vi "meth.PushClusterArray.vi"(0 "class.GLue in":refnum<class "class.GLue.lvclass">, 7 "Array":variant[](array[variant]), 11 "error in":errorcluster) -> (4 "class.GLue out":refnum<class "class.GLue.lvclass">, 8 "Pushed?":bool=TRUE, 15 "error out":errorcluster)   [LabVIEW 2014, in "GLue.lvlib" / "class.GLue.lvclass"]
uses:
  class.GLue.lvclass
  class.GLue.lvclass/class.GLue.ctl
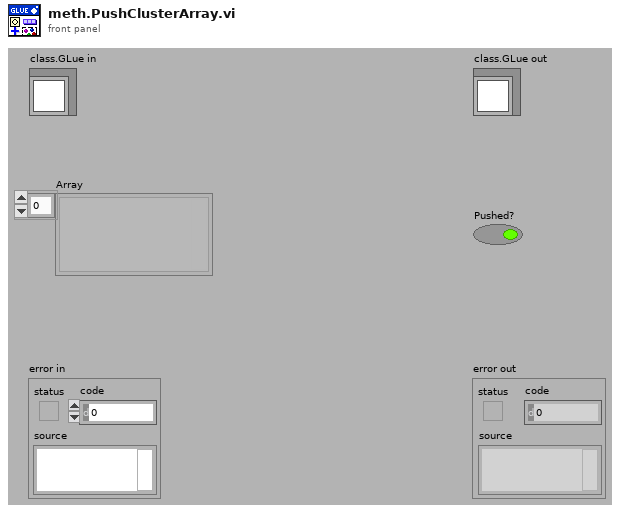
[diagram p1: front panel]
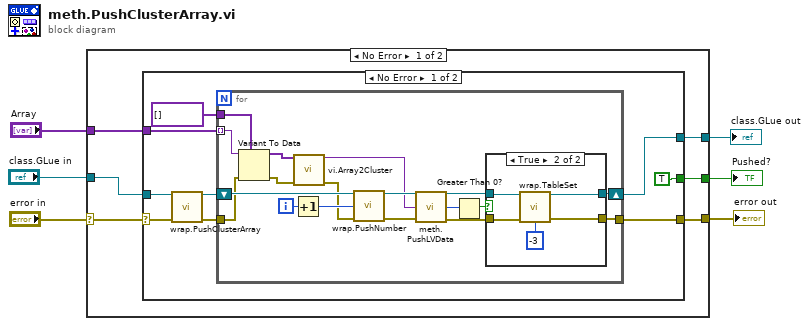
[diagram p0: block diagram]
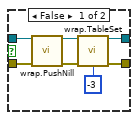
[diagram p2: hidden frame]
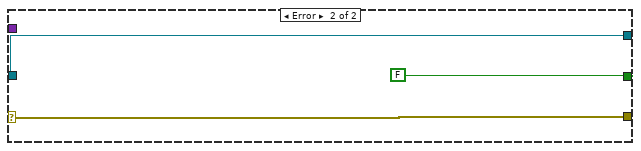
[diagram p4: hidden frame]
diagram:
  n1 = case shown="No Error" "error in" {
    selector: "error in" -> [w8 w57]
    tunnel: [w7 w57] -> w6
    tunnel: [w11 w56] -> w4
    tunnel: "class.GLue in" -> [w12 w56]
    tunnel: [w10 FALSE] -> w2
    tunnel: "Array" -> [w9 _]
    frame No Error {
      n2 = case shown="No Error" w8 {
        selector: w8 -> [w17 w54]
        tunnel: w9 -> [w21 _]
        tunnel: [w19 w54] -> w7
        tunnel: w12 -> [w16 w53]
        tunnel: [w20 w53] -> w11
        tunnel: [TRUE FALSE] -> w10
        frame No Error {
          n3 = call "wrap.PushClusterArray.vi"("class.GLue in"=w16, "error in (no error)"=w17) -> ("class.GLue out"=w15:refnum<class "class.GLue.lvclass">, "error out"=w14:errorcluster)  [unwired: 12 in]
          n4 = for {
            tunnel: w21 -> [w28] mode=indexing
            tunnel: w14 -> [w26]
            shift-right: [w35] -> w20
            shift-left: w15 -> [w32]
            tunnel: [w34] -> w19
            tunnel: variant[] [] -> [w27]
            i -> [w30]
            stop <- w34 stop-if-true
            n5 = Variant To Data(error in=w26, type=w27, Variant=w28) -> (data=w25:variant[], error out=w23:errorcluster)
            n6 = Increment(x=w30) -> (x+1=w29:i32)
            n7 = call "vi.Array2Cluster.vi"("Array"=w25, "error in (no error)"=w23) -> ("Cluster"=w24:variant, "error out"=w22:errorcluster)  [unwired: 12 in]
            n8 = call "wrap.PushNumber.vi"("class.GLue in"=w32, "Numeric"=w29, "error in (no error)"=w22) -> ("class.GLue out"=w31:refnum<class "class.GLue.lvclass">, "error out"=w33:errorcluster)  [unwired: 11 in]
            n9 = call "meth.PushLVData.vi"("class.GLue in"=w31, "variant in"=w24, "error in (no error)"=w33) -> ("class.GLue out"=w37:refnum<class "class.GLue.lvclass">, "NumPushed"=w39:i32, "error out"=w36:errorcluster)  [unwired: 10 in]
            n10 = Greater Than 0?(x=w39) -> (x > 0?=w38:bool)
            n11 = case shown="True" w38 {
              tunnel: w37 -> [w46 w50]
              tunnel: w36 -> [w45 w51]
              tunnel: [w41 w47] -> w34
              tunnel: [w40 w48] -> w35
              frame False {
                n12 = call "wrap.PushNill.vi"("class.GLue in"=w46, "error in (no error)"=w45) -> ("class.GLue out"=w42:refnum<class "class.GLue.lvclass">, "error out"=w43:errorcluster)  [unwired: 12 in]
                n13 = call "wrap.TableSet.vi"("class.GLue in"=w42, "error in (no error)"=w43, "Index"=-3) -> ("class.GLue out"=w40:refnum<class "class.GLue.lvclass">, "error out"=w41:errorcluster)  [unwired: 11 in]
              }
              frame True {
                n14 = call "wrap.TableSet.vi"("class.GLue in"=w50, "error in (no error)"=w51, "Index"=-3) -> ("class.GLue out"=w48:refnum<class "class.GLue.lvclass">, "error out"=w47:errorcluster)  [unwired: 11 in]
              }
            }
          }
        }
        frame Error {
        }
      }
    }
    frame Error {
    }
  }
  "error out" <- w6
  "class.GLue out" <- w4
  "Pushed?" <- w2
